vi "Write Position.vi"(8 "error in (no error)":errorcluster, 9 "Position":T1, 10 "VISA resource name in":refnum<visa-resource-name>, 11 "LCD-I2C in":refnum<class "LCD-I2C.lvclass">) -> (0 "error out":errorcluster, 2 "VISA resource name":refnum<visa-resource-name>, 3 "LCD-I2C out":refnum<class "LCD-I2C.lvclass">)   [LabVIEW 2020, in "CTI-Visa-DeviceLib.lvlib" / "LCD-I2C.lvclass"]
uses:
  LCD-I2C.lvclass
  Position.ctl
  Command.ctl
  LCD-I2C.lvclass/LCD-I2C.ctl
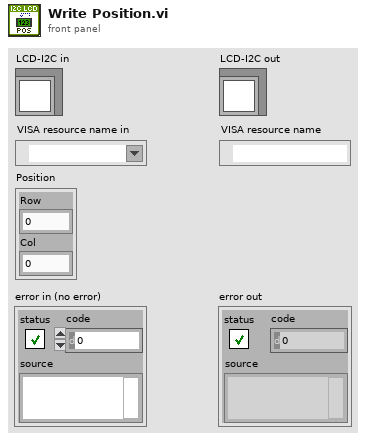
[diagram p1: front panel]
types:
  T1 = typedef "CTI-Visa-DeviceLib.lvlib/LCD-I2C.lvclass/Position.ctl" = cluster{"Row":u8, "Col":u8}
  T2 = typedef "CTI-Visa-DeviceLib.lvlib/LCD-I2C.lvclass/Command.ctl" = enum16{"Clear Display", "Return Home", "Entry Mode Set", "Display Control", "Cursor Shift", "Function Set", "Set CGRAM Addr", "Set DDRAM Addr"}
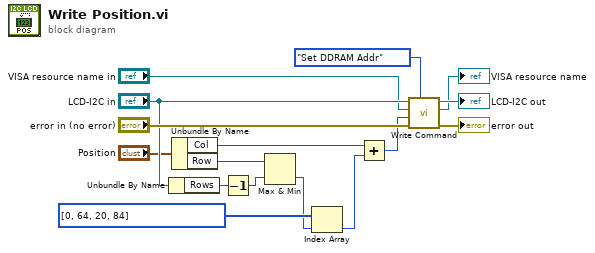
[diagram p0: block diagram]
diagram:
  n1 = Unbundle By Name("LCD-I2C in") -> ("Rows"=w11:u8)
  n2 = Unbundle By Name("Position") -> ("Col"=w6:u8, "Row"=w9:u8)
  n3 = Decrement(x=w11) -> (x-1=w1:u8)
  n4 = Max & Min(x=w9, y=w1) -> (min(x,y)=w7:u8)  [unwired: 1 out]
  n5 = Index Array(array=u8[] [0, 64, 20, 84], index=w7) -> (element=w5:u8)
  n6 = Add(x=w6, y=w5) -> (x+y=w4:u8)
  n7 = call "Write Command.vi"("Command"=Command."Set DDRAM Addr", "error in (no error)"="error in (no error)", "Value"=w4, "VISA resource name in"="VISA resource name in", "LCD-I2C in"="LCD-I2C in") -> ("error out"=→"error out":errorcluster, "VISA resource name"=→"VISA resource name":refnum<visa-resource-name>, "LCD-I2C out"=→"LCD-I2C out":refnum<class "LCD-I2C.lvclass">)  [unwired: 4 in]
